vi "daqio_Write_Multiple.vi"(7 "daq.io Device Channel Keys":string[](array[string]), 8 "error in (no error)":errorcluster, 9 "Timestamps":timestamp[](array[timestamp]), 10 "Values":dbl[](array[numeric]), 11 "daq.io type in":T1={"daq.io ref"=refnum, "daq.io API Base"="http://dashboard.daq.io/api/v1", "Device Key"="", "Account ID"="", "online"=TRUE, "SSL"=FALSE}) -> (0 "error out":errorcluster, 3 "daq.io type out":T1={"daq.io ref"=refnum, "daq.io API Base"="http://dashboard.daq.io/api/v1", "Device Key"="", "Account ID"="", "online"=TRUE, "SSL"=FALSE})   [LabVIEW 2013, in "daqio minimal.lvlib"]
doc: "This VI writes multiple data points to a channel of a daq.io device. \n\nIf the daq.io Device Channel does not exist online, a new channel will be auto-created and data will be stored there. You have to provide a Channel Key where the value will be written to."
uses:
  daqio minimal.lvlib
  _typedefs/daqio-Type.ctl
  <vilib>/httpClient/ClientHandle.ctl
  _typedefs/daqio-TimeSeriesEntry.ctl
  _typedefs/daqio-Buffer-Commands.ctl
  _typedefs/connection_FGV_commands.ctl
  <vilib>/Easy HTTP Client/Easy HTTP.lvlib
  <vilib>/httpClient/LabVIEWHTTPClient.lvlib
panel:
  out "JSON string":string
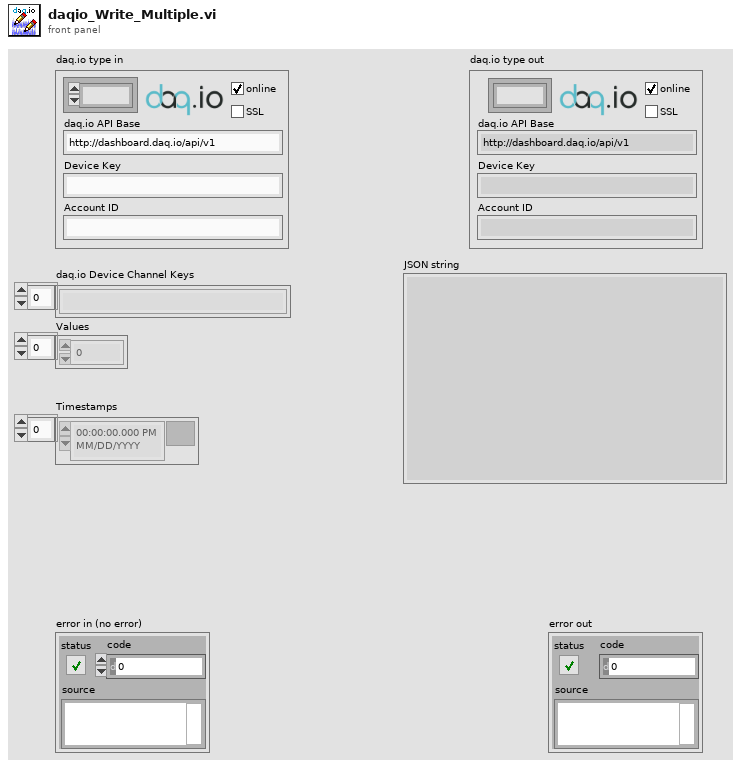
[diagram p1: front panel]
types:
  T1 = typedef "daqio minimal.lvlib/daqio-Type.ctl" = cluster{"daq.io ref":T2, "daq.io API Base":string, "Device Key":string, "Account ID":string, "online":bool, "SSL":bool}
  T2 = typedef "LabVIEWHTTPClient.lvlib/ClientHandle.ctl" = refnum<k1>
  T3 = typedef "daqio minimal.lvlib/daqio-TimeSeriesEntry.ctl" = cluster{"channel":string, "time":string, "value":dbl}
  T4 = typedef "daqio minimal.lvlib/daqio-Buffer-Commands.ctl" = enum16{"Add to Buffer", "Post from Buffer", "Clear Buffer", "Init"}
  T5 = typedef "daqio minimal.lvlib/connection_FGV_commands.ctl" = enum16{"Set Conn Stat", "Save Type", "Get Type from File", "Set Type", "Set Buffer", "Get"}
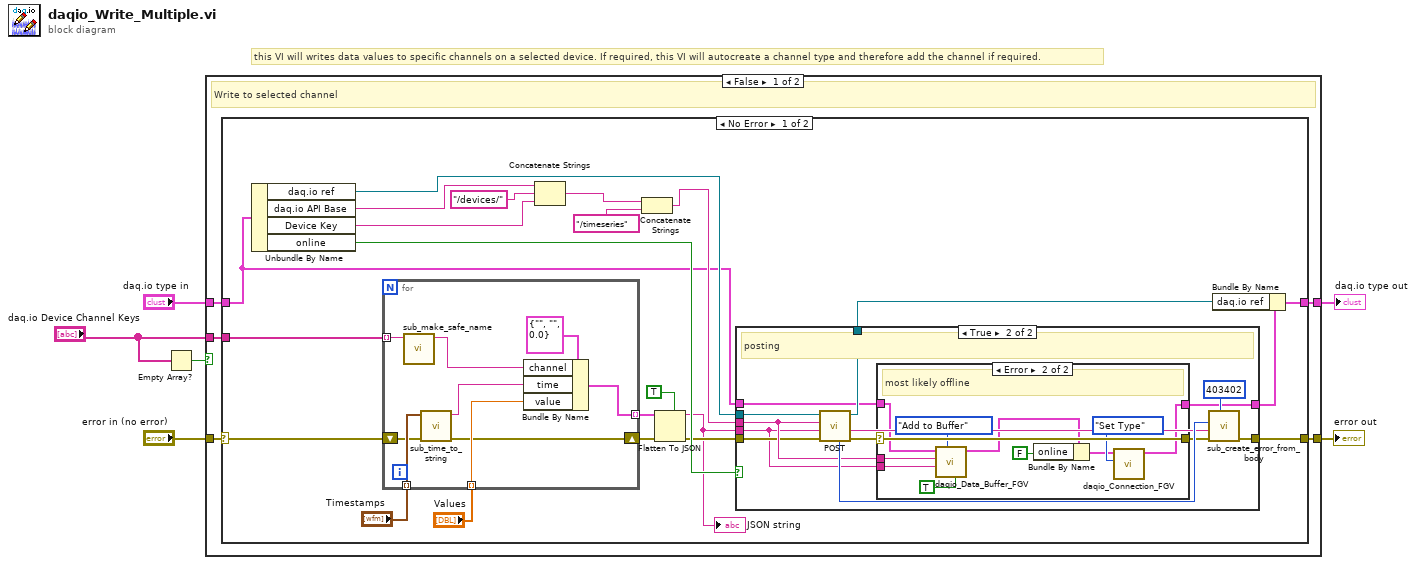
[diagram p0: block diagram]
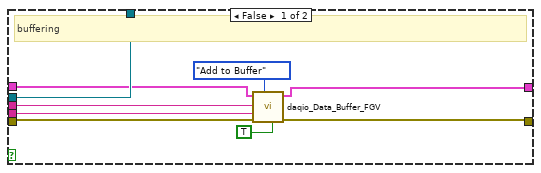
[diagram p2: hidden frame]
diagram:
  # "this VI will writes data values to specific channels on a selected device. If required, this VI will autocreate a channel type and therefore add the channel if required."
  n1 = Empty Array?(array="daq.io Device Channel Keys") -> (empty?=w3:bool)
  n2 = case shown="False" w3 {
    tunnel: "daq.io type in" -> [w11 w81]
    tunnel: [w10 w81] -> w6
    tunnel: [w9 w80] -> w5
    tunnel: "error in (no error)" -> [w8 w80]
    tunnel: "daq.io Device Channel Keys" -> [w7 _]
    frame False {
      # "Write to selected channel"
      n3 = case shown="No Error" w8 {
        selector: w8 -> [w25 w78]
        tunnel: w11 -> [w12 w79]
        tunnel: [w16 w79] -> w10
        tunnel: [w26 w78] -> w9
        tunnel: w7 -> [w27 _]
        frame No Error {
          n4 = Unbundle By Name(w12) -> ("daq.io ref"=w28:T2, "daq.io API Base"=w33:string, "Device Key"=w13:string, "online"=w24:bool)
          n5 = for {
            tunnel: w27 -> [w35] mode=indexing
            shift-right: [w37] -> w20
            shift-left: w25 -> [w36]
            tunnel: "Timestamps" -> [w42] mode=indexing
            tunnel: "Values" -> [w41] mode=indexing
            tunnel: [w38] -> w21 mode=indexing
            n6 = call "sub_make_safe_name.vi"("Input String"=w35) -> ("Safe Output String"=w34:string)  [unwired: 10 in]
            n7 = call "sub_time_to_string.vi"("error in (no error)"=w36, "timestamp"=w42) -> ("error out"=w37:errorcluster, "time"=w40:string)  [unwired: 8 in]
            n8 = Bundle By Name(cluster=T3 {"channel"="", "time"="", "value"=0.0}, "channel"=w34, "time"=w40, "value"=w41) -> (w38:T3)
          }
          n9 = Concatenate Strings(w33, "/devices/", w13) -> (w29:string)
          n10 = Concatenate Strings(w29, "/timeseries") -> (w30:string)
          n11 = Flatten To JSON(enable LabVIEW extensions? (T)=TRUE, anything=w21, error in (no error)=w20) -> (JSON string=w17:string, 11:w18:errorcluster)
          "JSON string" <- w17
          n12 = case shown="True" w24 {
            tunnel: [w51 w64] -> w32
            tunnel: w30 -> [w49 w55]
            tunnel: w28 -> [w51 w63]
            tunnel: [w50 w62] -> w26
            tunnel: w12 -> [w47 w57]
            tunnel: [w45 w56] -> w15
            tunnel: w18 -> [w44 w53]
            tunnel: w17 -> [w46 w52]
            frame False {
              # "buffering"
              n13 = call "daqio_Data_Buffer_FGV.vi"("Is Array?"=TRUE, "Buffer Command"=daqio-Buffer-Commands."Add to Buffer", "error in (no error)"=w44, "JSON Data"=w46, "API route"=w49, "daq.io type in"=w47) -> ("error out"=w50:errorcluster, "daq.io type out"=w45:T1)  [unwired: 4 in]
            }
            frame True {
              # "posting"
              n14 = call <vilib>:"POST.vi"("error in (no error)"=w53, "data"=w52, "url"=w55, "client handle"=w63) -> ("error out"=w58:errorcluster, "body"=w59:string, "client handle out"=w64:T2, "HTTP Response Code"=w61:i32)  [unwired: 3 in, 1 out]
              n15 = case shown="Error" w58 {
                selector: w58 -> [w66 w77]
                tunnel: [w66 w77] -> w54
                tunnel: [w65 w67] -> w56
                tunnel: w57 -> [w65 w68]
                tunnel: w55 -> [_ w71]
                tunnel: w52 -> [_ w70]
                frame No Error {
                }
                frame Error {
                  # "most likely offline"
                  n16 = call "daqio_Data_Buffer_FGV.vi"("Is Array?"=TRUE, "Buffer Command"=daqio-Buffer-Commands."Add to Buffer", "JSON Data"=w70, "API route"=w71, "daq.io type in"=w68) -> ("daq.io type out"=w74:T1)  [unwired: 5 in, 1 out]
                  n17 = Bundle By Name(cluster=w74, "online"=FALSE) -> (w72:T1)
                  n18 = call "daqio_Connection_FGV.vi"("Enum"=connection_FGV_commands."Set Type", "daq.io type in"=w72) -> ("daq.io type out"=w67:T1)  [unwired: 6 in, 3 out]
                }
              }
              n19 = call "sub_create_error_from_body.vi"("error code"=403402, "error in (no error)"=w54, "http code"=w61, "body"=w59) -> ("error out"=w62:errorcluster)  [unwired: 7 in]
            }
          }
          n20 = Bundle By Name(cluster=w15, "daq.io ref"=w32) -> (w16:T1)
        }
        frame Error {
        }
      }
    }
    frame True {
      # "no Channel Key: nothing to do"
    }
  }
  "error out" <- w5
  "daq.io type out" <- w6
